vi "Initiate Dispense.vi"(8 "error in (no error)":errorcluster, 11 "VISA resource name":refnum<visa-resource-name>) -> (0 "error out":errorcluster, 3 "VISA resource name out":refnum<visa-resource-name>)   [LabVIEW 2016, in "EFD Ultimus V.lvlib"]
doc: "Initiates a dispense cycle in the Ultimus V. If the unit is in timed mode, the unit will dispense for the duration currently set in dispense time parameter. If the unit is in steady mode, the unit will begin dispensing. Another dispense command is then needed to end the dispense cycle. \n\nHost Format: DI--"
uses:
  EFD Ultimus V.lvlib
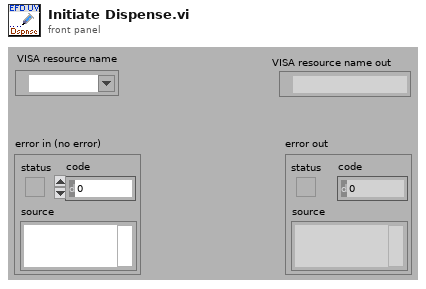
[diagram p1: front panel]
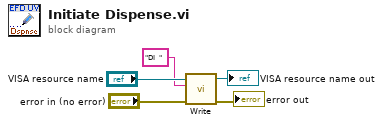
[diagram p0: block diagram]
diagram:
  n1 = call "Write.vi"("error in (no error)"="error in (no error)", "Command To Write"="DI  ", "VISA resource name"="VISA resource name") -> ("error out"=→"error out":errorcluster, "VISA resource name out"=→"VISA resource name out":refnum<visa-resource-name>)  [unwired: 7 in]
